vi "GetTrigger.vi"(7 "ModuleID":i32, 8 "error in (no error)":errorcluster, 11 "IVI_Class in":refnum<class "IVI_Class.lvclass">) -> (0 "error out":errorcluster, 3 "IVI_Class out":refnum<class "IVI_Class.lvclass">)   [LabVIEW 2018, in "ScopePlugins.lvlib" / "IVI_Class.lvclass"]
uses:
  IVI_Class.lvclass
  ScopePluginBaseClass/ScopePluginsBase.lvclass
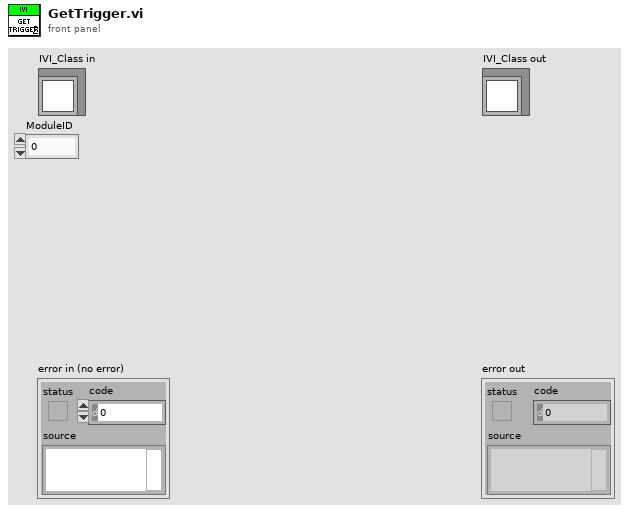
[diagram p1: front panel]
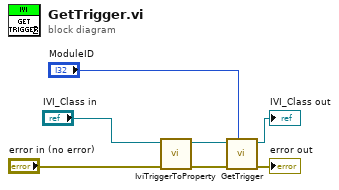
[diagram p0: block diagram]
diagram:
  n1 = call "IviTriggerToProperty.vi"("error in (no error)"="error in (no error)", "IVI_Class.lvclass"="IVI_Class in") -> ("error out"=w1:errorcluster, "IVI_Class.lvclass"=w2:refnum<class "IVI_Class.lvclass">)  [unwired: 8 in]
  n2 = call-parent "GetTrigger.vi"("ModuleID"="ModuleID", "error in (no error)"=w1, "ScopePluginsBase in"=w2) -> ("error out"=→"error out":errorcluster, "ScopePluginsBase out"=→"IVI_Class out":refnum<class "IVI_Class.lvclass">)  [unwired: 7 in]
